vi "Handle Error.vi"(8 "error in (no error)":errorcluster, 11 "UI ActorTop in":refnum<class "Model_AMC.lvclass">) -> (0 "error out":errorcluster, 2 "stop actor?":bool=TRUE, 3 "UI ActorTop out":refnum<class "Model_AMC.lvclass">)   [LabVIEW 2021, in "Model_AMC.lvclass"]
doc: "(<B>Filename</B>: Actor Framework.lvlib:Actor.lvclass:Handle Error.vi)\n\nDefines how the actor handles an error that occurred while processing a message. By default, this method does nothing except stop the actor."
uses:
  Model_AMC.lvclass
  <userlib>/John_Lib/AbstractActorTemplate/AbstractActorTemplate/UIActorTop.lvclass
  Model_AMC.lvclass/Model_AMC.ctl
  <vilib>/ActorFramework/Stop Msg/Stop Msg.lvclass
  b9e01822-7322-460e-95c5-51048fa5dd75.vi
  C:/Program Files (x86)/National Instruments/LabVIEW 2021/user.lib/John_Lib/AbstractActorTemplate/AbstractActorTemplate/UIActorTop.lvclass
  C:/Program Files (x86)/National Instruments/LabVIEW 2021/vi.lib/ActorFramework/Actor/Actor.lvclass
  C:/Program Files (x86)/National Instruments/LabVIEW 2021/project/Create Actor from Template/_Model_AMC/Model_AMC.lvclass
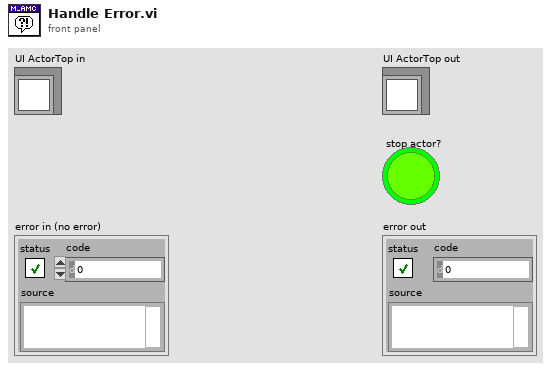
[diagram p1: front panel]
types:
  T1 = map{string, refnum<class "Message Enqueuer.lvclass">}
  T2 = typedef "AMC_FW.lvlib/Queue.ctl" = cluster{"Q":T3, "Name":string}
  T3 = typedef "AMC_FW.lvlib/Message Queue.ctl" = refnum<queue>
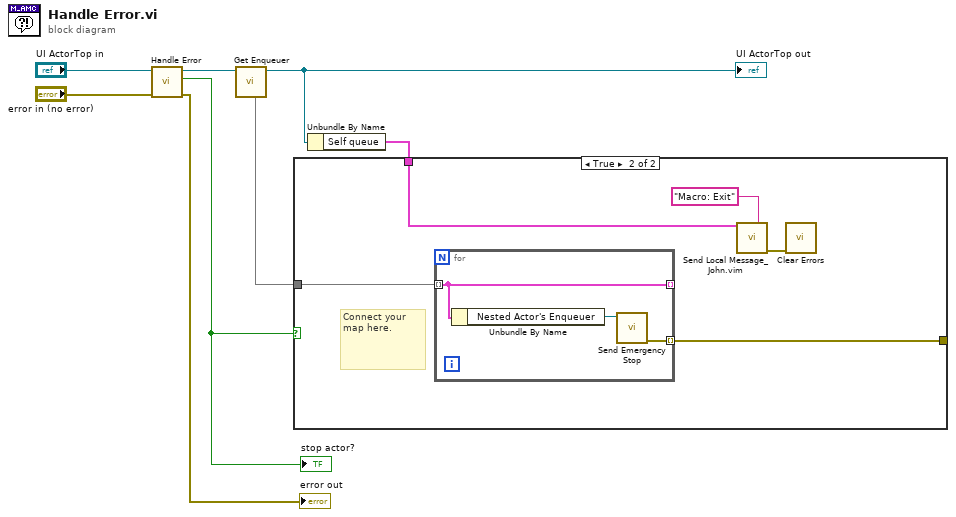
[diagram p0: block diagram]
diagram:
  n1 = call-parent "Handle Error.vi"("error in (no error)"="error in (no error)", "UI ActorTop in"="UI ActorTop in") -> ("error out"=→"error out":errorcluster, "stop actor?"=w4:bool, "UI ActorTop out"=w3:refnum<class "Model_AMC.lvclass">)  [unwired: 7 in]
  "stop actor?" <- w4
  n2 = call <userlib>:"Get Enqueuer.vi"("UIActorTop in"=w3) -> ("UIActorTop out"=w1:refnum<class "Model_AMC.lvclass">, "Enqueuer"=w5:T1)  [unwired: 4 in, 5 out]
  "UI ActorTop out" <- w1
  n3 = Unbundle By Name(w1) -> ("Self queue"=w2:T2)
  n4 = case shown="True" w4 {
    tunnel: w5 -> [_ w13]
    tunnel: [_ w12] -> _
    tunnel: w2 -> [_ w9]
    frame False {
    }
    frame True {
      # "Connect your map here."
      n5 = for {
        tunnel: [w16] -> _ mode=indexing
        tunnel: w13 -> [w16] mode=indexing
        tunnel: [w14] -> w12 mode=indexing
        n6 = Unbundle By Name(w16) -> ("Nested Actor's Enqueuer"=w15:refnum<class "Message Enqueuer.lvclass">)
        n7 = call <vilib>:"Send Emergency Stop.vi"("Message Enqueuer"=w15) -> ("error out"=w14:errorcluster)  [unwired: 10 in]
      }
      n8 = call "Send Local Message_John.vim"("Queue In"=w9, "Elements in Front"="Macro: Exit") -> ("error out"=w10:errorcluster)  [unwired: 11 in, 2 out]
      n9 = call <vilib>:"Clear Errors.vi"("error in (no error)"=w10) -> ()  [unwired: 5 in, 2 out]
    }
  }
